vi "Read With Abort.vi"(7 "timeout in ms (-1)":i32=-1, 9 "abort":bool, 10 "channel":T1) -> (1 "last element?":bool, 2 "element":T2, 3 "element valid?":bool, 4 "aborted?":bool, 5 "timed out?":bool, 6 "count":i32)   [LabVIEW 2017, in "Stream-t'WPI_EncoderType.ctl'.lvlib"]
doc: "Reads an element from a Stream channel or signals the channel to abort. This endpoint is the same as the Read endpoint except that it has an <B>abort</B> input and an <B>aborted?</B> output. You can use the abort capability of the Stream channel to close a channel abruptly, ignoring any data left in the channel buffer. You must use this endpoint together with the Write With Abort endpoint."
uses:
  <extravilib>/ChannelInstances/Stream-t'WPI_EncoderType.ctl'.lvlib
  <vilib>/Rock Robotics/WPI/Encoder/WPI_EncoderType.ctl
  <extravilib>/ChannelInstances/Stream-t'WPI_EncoderType.ctl'/)Channel.ctl
  <resource>/ChannelSupport/_ChannelSupport/WaitIfNeeded.vi
  <extravilib>/ChannelInstances/Stream-t'WPI_EncoderType.ctl'/)Channel.vi
panel:
  # "legal combinations:\n    aborted\n    timedout\n    valid\n    valid, last element\n    last element"
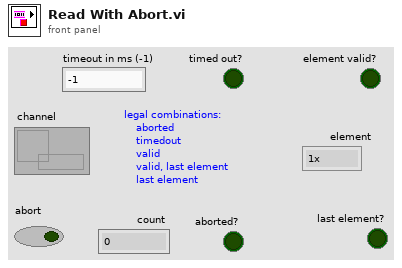
[diagram p1: front panel]
types:
  T1 = typedef "Stream-t'WPI_EncoderType.ctl'.lvlib/)Channel.ctl" = refnum<queue>
  T2 = typedef "WPI_EncoderType.ctl" = enum16{"1x", "2x", "4x"}
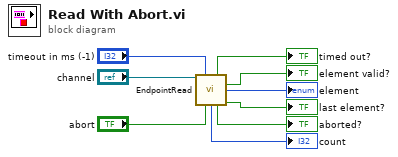
[diagram p0: block diagram]
diagram:
  n1 = call <extravilib>:"EndpointRead.vi"("channel in"="channel", "timeout in ms (-1)"="timeout in ms (-1)", "abort (F)"="abort") -> ("timed out?"=→"timed out?":bool, "valid?"=→"element valid?":bool, "element out"=→"element":T2, "count"=→"count":i32, "aborted?"=→"aborted?":bool, "last element?"=→"last element?":bool)  [unwired: 7 in]
